vi "relays.vi"() -> ()   [LabVIEW 2025]
uses:
  <vilib>/DAQmx/create/channels.llb/DAQmx Create Channel (DO-Digital Output).vi
  <vilib>/DAQmx/write.llb/DAQmx Write (Digital Bool 1Line 1Point).vi
  <vilib>/DAQmx/create/channels.llb/DAQmx Create Channel (AI-Temperature-Thermocouple).vi
panel:
  out "task out":refnum<k21>
  in  "Delay Time (s)":dbl=1.0
  out "error out":errorcluster
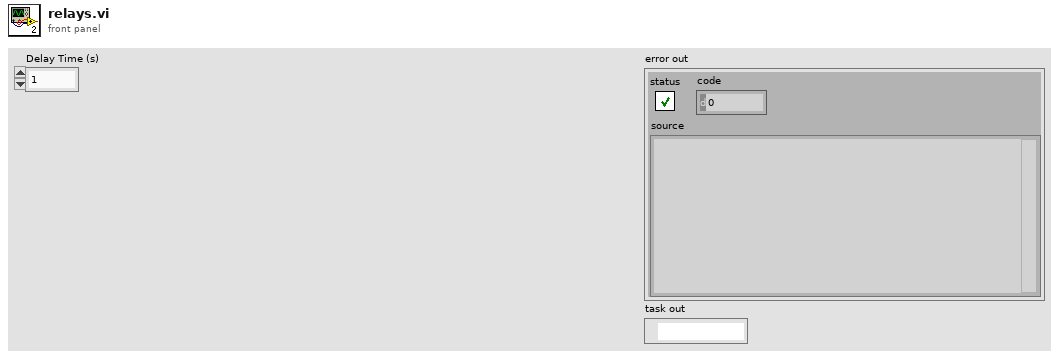
[diagram p1: front panel]
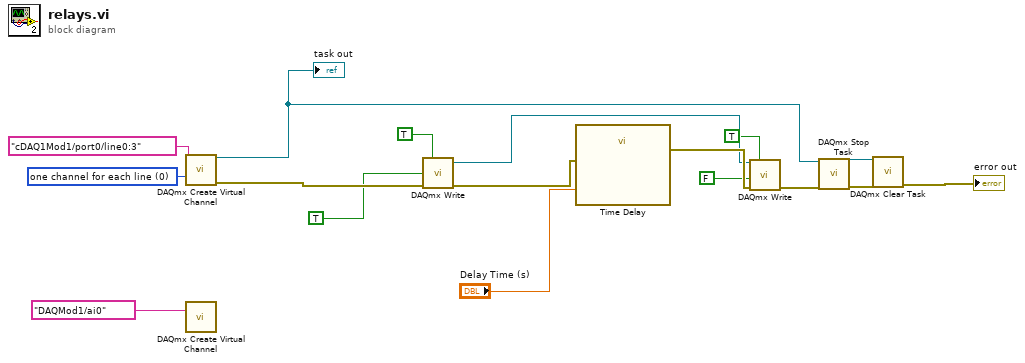
[diagram p0: block diagram]
diagram:
  w5 = 0 items=["one channel for each line", "one channel for all lines"] ("line grouping")
  n1 = call-poly <vilib>:"DAQmx Create Virtual Channel.vi"("lines"=tag "cDAQ1Mod1/port0/line0:3", "line grouping"=w5) -> ("task out"=w2:refnum<k21>, "error out"=w4:errorcluster)  [unwired: 12 in]
  "task out" <- w2
  n2 = call-poly <vilib>:"DAQmx Create Virtual Channel.vi"("physical channels"=tag "DAQMod1/ai0") -> ()  [unwired: 13 in, 2 out]
  n3 = call-poly <vilib>:"DAQmx Write.vi"("auto start"=TRUE, "data"=TRUE, "error in"=w4) -> ("task out"=w14:refnum<k21>, "error out"=w16:errorcluster)  [unwired: 10 in, 1 out]
  n4 = call "Time Delay"("error in (no error)"=w16, "Delay Time (s)"="Delay Time (s)") -> ("error out"=w15:errorcluster)  [unwired: 9 in]
  n5 = call-poly <vilib>:"DAQmx Write.vi"("task/channels in"=w14, "auto start"=TRUE, "data"=FALSE, "error in"=w15) -> ("error out"=w12:errorcluster)  [unwired: 9 in, 2 out]
  n6 = call <vilib>:"DAQmx Stop Task.vi"("task/channels in"=w2, "error in"=w12) -> ("task out"=w11:refnum<k21>, "error out"=w10:errorcluster)  [unwired: 12 in]
  n7 = call <vilib>:"DAQmx Clear Task.vi"("task in"=w11, "error in"=w10) -> ("error out"=→"error out":errorcluster)  [unwired: 13 in]
